vi "PID_Velocity.vi"() -> ()   [LabVIEW 2017]
uses:
  <vilib>/Platform/TimedLoop/XDataNode/timing_clust.ctl
  <vilib>/Platform/TimedLoop/XDataNode/nitl_modes.ctl
  <vilib>/Platform/TimedLoop/XDataNode/wakeup.ctl
  <vilib>/myRIO/Instrument Drivers/Onboard IO/AO/typedefs/AO Reference.ctl
  <vilib>/myRIO/Common/Instrument Driver Framework/Utilities/typedefs/myRIO Generic Hardware Reference.ctl
  <vilib>/myRIO/Common/Instrument Driver Framework/Utilities/typedefs/Hardware Version Enum.ctl
  <vilib>/myRIO/Common/Instrument Driver Framework/Utilities/typedefs/myRIO v1.0 Reference.ctl
  <vilib>/myRIO/Common/Instrument Driver Framework/Utilities/typedefs/Generic FPGA Reference.ctl
  <vilib>/myRIO/Common/Instrument Driver Framework/myRIO v1.0/AO/typedefs/AO Channels List.ctl
  <vilib>/myRIO/Common/Instrument Driver Framework/myRIO v1.0/AO/typedefs/AO Channels Enum.ctl
  <vilib>/myRIO/Common/Instrument Driver Framework/Utilities/typedefs/Analog Scaling Constants List.ctl
  <vilib>/myRIO/Common/Instrument Driver Framework/Utilities/typedefs/Analog Scaling Constants.ctl
  <vilib>/userdefined/High Color/nirio_resource_hc.ctl
  <vilib>/myRIO/Common/Instrument Driver Framework/Utilities/vis/Is FPGA Ref Available.vi
  <vilib>/myRIO/Common/Instrument Driver Framework/myRIO v1.0/AO/vis/myRIO v1.1 Open AO.vi
  <vilib>/myRIO/Instrument Drivers/Onboard IO/AO/vis/Write.vi
  <vilib>/myRIO/Common/Instrument Driver Framework/Utilities/vis/Validate Channels.vi
  <vilib>/myRIO/Common/Instrument Driver Framework/myRIO v1.0/AO/vis/myRIO v1.0 Reserve AO.vi
  <vilib>/myRIO/Common/Instrument Driver Framework/myRIO v1.0/AO/vis/myRIO v1.0 Build MUX Configuration AO.vi
  <vilib>/myRIO/Common/Instrument Driver Framework/myRIO v1.0/Resource Manager/vis/myRIO v1.0 Reserve Channel List.vi
  <vilib>/myRIO/Common/Instrument Driver Framework/myRIO v1.0/Resource Manager/vis/myRIO v1.0 Reserve Channel.vi
  <vilib>/myRIO/Common/Instrument Driver Framework/myRIO v1.0/Resource Manager/vis/myRIO v1.0 Unreserve Channel.vi
  <vilib>/myRIO/Common/Instrument Driver Framework/myRIO v1.0/Resource Manager/vis/myRIO v1.0 Build Mutex Name.vi
  <vilib>/Utility/VariantDataType/GetNumericInfo.vi
  <vilib>/Utility/error.llb/Error Cluster From Error Code.vi
  <vilib>/myRIO/Common/Instrument Driver Framework/myRIO v1.0/myRIO v1.1 Open.vi
  <vilib>/myRIO/Common/Instrument Driver Framework/myRIO v1.0/AO/vis/myRIO v1.0 Get Scaling Constants AO.vi
  <vilib>/myRIO/Common/Instrument Driver Framework/Utilities/vis/IO Manager.vi
  <vilib>/myRIO/Common/Instrument Driver Framework/Utilities/vis/Configuration Manager.vi
  <vilib>/myRIO/Common/Instrument Driver Framework/myRIO v1.0/myRIO v1.0 Close.vi
  <vilib>/myRIO/Common/Instrument Driver Framework/myRIO v1.0/AO/vis/myRIO v1.0 Write AO.vi
  <vilib>/addons/control/pid/pid.llb/PID (DBL).vi
  <vilib>/platform/TimedLoop/XDataNode/XDataNode.xnode
  <vilib>/myRIO/Express VI/Onboard IO/AO/AO Express VI.xnode
  <vilib>/myRIO/Instrument Drivers/Onboard IO/AO/vis/myRIO AO Open.xnode
  <vilib>/addons/control/pid/NI_PID_pid.lvlib
  <vilib>/myRIO/Instrument Drivers/Onboard IO/AO/AO.lvlib
  <vilib>/Platform/TimedLoop/XDataNode/XDNodeRunTimeDep.lvlib
panel:
  out "Velocity":dbl(graph)
  out "Theta Rate (deg/s)":dbl
  out "error out":errorcluster
  out "process variable":dbl
  out "Setpoint":dbl
  out "analog output":dbl format="%.2f"
  in  "PID Range":cluster{"output high":dbl, "output low":dbl}={"output high"=3.2, "output low"=1.8} {"output low" format="%.2f"; "output high" format="%.2f"}
  in  "PID gains":T1={"proportional gain (Kc)"=2.0, "integral time (Ti, min)"=0.05, "derivative time (Td, min)"=0.0} {"derivative time (Td, min)" format="%.3f"; "integral time (Ti, min)" format="%.3f"; "proportional gain (Kc)" format="%.3f"}
  out "Position":cluster{"setpoint":dbl, dbl}(graph)={"setpoint"=303.908879655711, 0.0}
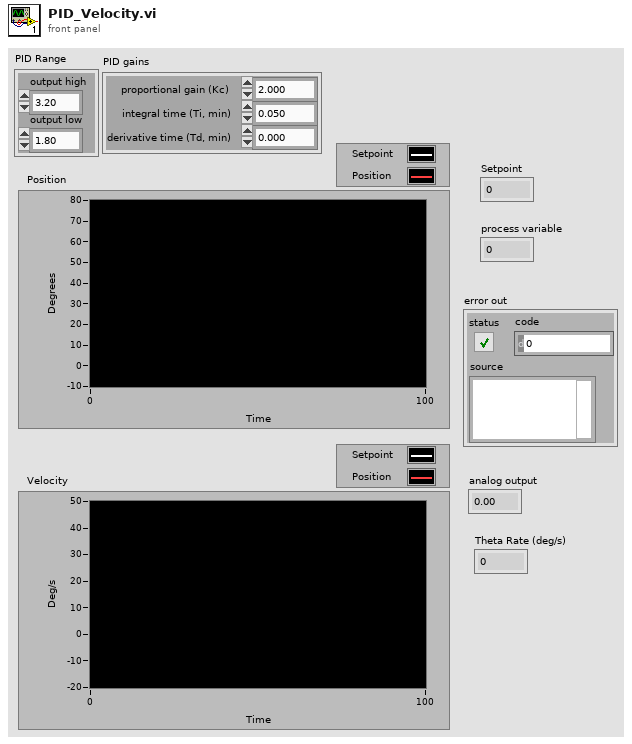
[diagram p1: front panel]
types:
  T1 = cluster{"proportional gain (Kc)":dbl, "integral time (Ti, min)":dbl, "derivative time (Td, min)":dbl}
  T2 = typedef "AO.lvlib/AO Reference.ctl" = cluster{"myRIO Reference":T3, "AO Channel List":T7, "AO Scaling Constant List":T9}
  T3 = typedef "myRIO Generic Hardware Reference.ctl" = cluster{"myRIO Model":T4, "myRIO Hardware Reference":T5}
  T4 = typedef "Hardware Version Enum.ctl" = enum16{"Unknown", "myRIO-1900", "myRIO-1950", "roboRIO", "NI ELVIS RIO CM"}
  T5 = typedef "myRIO v1.0 Reference.ctl" = cluster{"Generic FPGA Reference":T6, "Allow multiple opens":bool}
  T6 = typedef "Generic FPGA Reference.ctl" = refnum<k20>
  T7 = typedef "AO Channels List.ctl" = T8[]
  T8 = typedef "AO Channels Enum.ctl" = enum16{"Not Connected", "AudioOut/Left", "AudioOut/Right", "C/AO0", "C/AO1", "A/AO0", "A/AO1", "B/AO0", "B/AO1"}
  T9 = typedef "Analog Scaling Constants List.ctl" = T10[]
  T10 = typedef "Analog Scaling Constants.ctl" = cluster{"LSB Weight (Volts)":dbl, "Offset (Volts)":dbl, "Signed?":bool}
  T11 = typedef "nirio_resource_hc.ctl" = tag
  T12 = typedef "XDNodeRunTimeDep.lvlib/timing_clust.ctl" = cluster{"Expected End [f-1]":u64, "Actual End [f-1]":u64, "Finished Late? [f-1]":bool, "Expected End [i-1]":u64, "Actual End [i-1]":u64, "Finished Late? [i-1]":bool, "Expected Start [i]":u64, "Actual Start [i]":u64, "Expected Start [f]":u64, "Actual Start [f]":u64, "Source Name":string, "Structure Name":string, "Period":i64, "Deadline":i64, "Offset":i64, "Start":i64, "Priority":i32, "Timeout":i32, "Mode":T13, "Wakeup Reason":T14, "Error":errorcluster, "Source Type":string, "Secondary Source Type":string, "Global End Time":u64, "Global Start Time":u64, "Frame Duration":u64, "Iteration Duration":u64, "Assigned CPU":i32, "I/O Scan Engine Mode":u32}
  T13 = typedef "XDNodeRunTimeDep.lvlib/nitl_modes.ctl" = enum32{"No Change", "Process missed periods, maintain original phase", "Discard missed periods, maintain original phase", "Process missed periods, ignore original phase", "Discard missed periods, ignore original phase"}
  T14 = typedef "XDNodeRunTimeDep.lvlib/wakeup.ctl" = enum32{"Normal", "Aborted", "Asynchronous wakeup", "Timing source error", "Timed loop error", "Timeout"}
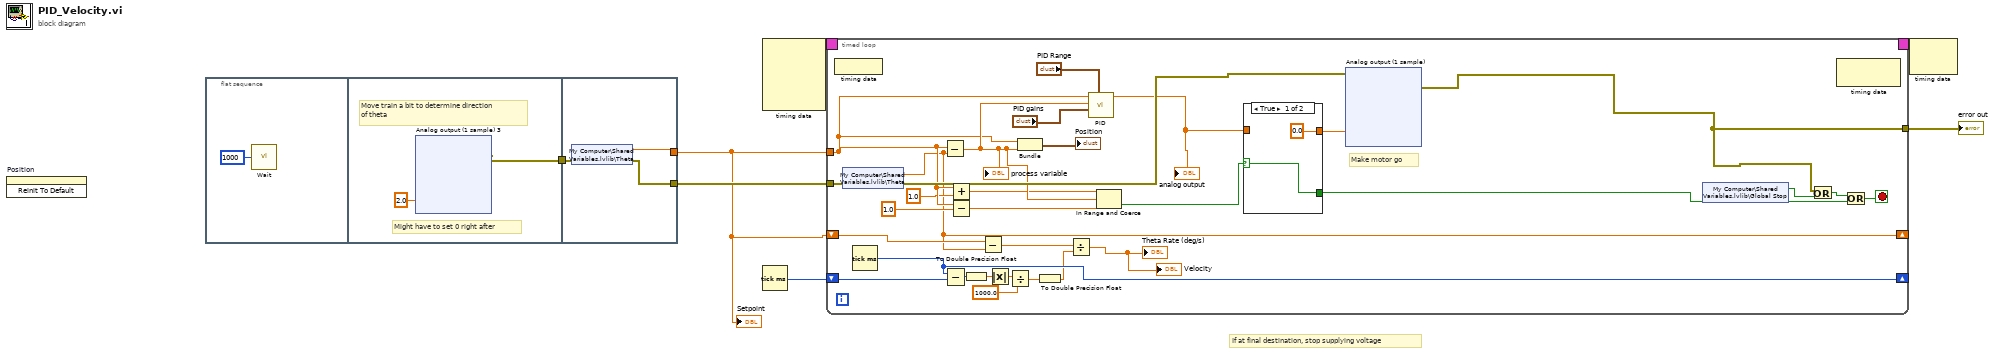
[diagram p0: block diagram]
diagram:
  # "If at final destination, stop supplying voltage"
  n1 = invoke on="Position" class="WFChart (strict)" method="Reinit To Default"() -> ()  [unwired: 3 in, 3 out]
  n2 = flat-sequence {
    tunnel: [w9] -> w3
    tunnel: [w50] -> w2
    tunnel: [w49] -> w5
    tunnel: w3 -> [w48]
    frame #0 {
      n3 = call "Wait"("Count(mSec)"=u32 1000) -> ()  [unwired: 1 out]
    }
    frame #1 {
      # "Might have to set 0 right after"
      # "Move train a bit to determine direction\nof theta"
      n4 = xnode "Analog output (1 sample) 3"("C/AO0 (AO0)"=2.0) -> ("error out"=w9:errorcluster)  [unwired: 1 in]
    }
    frame #2 {
      n5 = shared-variable "My Computer\\Shared Variables.lvlib\\Theta"(error in=w48) -> (w50:dbl, error out=w49:errorcluster)
    }
  }
  n6 = node-c288() -> (w7:T12)  [unwired: 4 in]
  n7 = Tick Count (ms)() -> (millisecond timer value=w1:u32)
  n8 = timed-loop {
    timing: w7 -> [_]
    timing-out: [_] -> w6
    tunnel: w2 -> [w75]
    tunnel: w5 -> [w78]
    tunnel: [w63] -> w4
    shift-right: [w51] -> _
    shift-left: w2 -> [w52]
    shift-right: [w61] -> _
    shift-left: w1 -> [w60]
    stop <- w65 stop-if-true
    # "Make motor go"
    n9 = node-c288() -> ()  [unwired: 1 in]
    n10 = shared-variable "My Computer\\Shared Variables.lvlib\\Theta"(error in=w78) -> (w51:dbl, error out=w77:errorcluster)
    n11 = Tick Count (ms)() -> (millisecond timer value=w61:u32)
    n12 = Subtract(x=w75, y=w51) -> (x-y=w76:dbl)
    "process variable" <- w76
    n13 = Subtract(x=w61, y=w60) -> (x-y=w56:u32)
    n14 = Add(x=w75, y=1.0) -> (x+y=w72:dbl)
    n15 = Subtract(x=w75, y=1.0) -> (x-y=w71:dbl)
    n16 = To Double Precision Float(number=w56) -> (double precision float=w55:dbl)
    n17 = Subtract(x=w52, y=w51) -> (x-y=w62:dbl)
    n18 = Absolute Value(x=w55) -> (abs(x)=w54:dbl)
    n19 = Divide(x=w54, y=1000.0) -> (x/y=w57:dbl)
    n20 = Bundle("Double"=w75, w76) -> (→"Position":cluster{"Double":dbl, dbl})  [unwired: 1 in]
    n21 = To Double Precision Float(number=w57) -> (double precision float=w59:dbl)
    n22 = Divide(x=w62, y=w59) -> (x/y=→"Theta Rate (deg/s)" →"Velocity":dbl)
    n23 = call-poly <vilib>:"PID.vi"("output range"="PID Range", "PID gains"="PID gains", "process variable"=w76, "setpoint"=w75) -> ("output"=w69:dbl)  [unwired: 6 in, 1 out]
    "analog output" <- w69
    n24 = In Range and Coerce(upper limit=w72, x=w76, lower limit=w71) -> (In Range?=w70:bool)  [unwired: 1 out]
    n25 = case shown="True" w70 {
      selector: w70 -> [w82 w84]
      tunnel: [0.0 ("output") w85] -> w68
      tunnel: w69 -> [_ w85]
      tunnel: [w82 w84] -> w67
      frame True {
      }
      frame False {
      }
    }
    n26 = xnode "Analog output (1 sample)"("C/AO0 (AO0)"=w68, "error in (no error)"=w77) -> ("error out"=w63:errorcluster)
    n27 = shared-variable "My Computer\\Shared Variables.lvlib\\Global Stop"() -> (w64:bool)  [unwired: 1 in, 1 out]
    n28 = Or(x=w63, y=w64) -> (x .or. y?=w66:bool)
    n29 = node-c288() -> ()  [unwired: 1 in, 1 out]
    n30 = Or(x=w66, y=w67) -> (x .or. y?=w65:bool)
  }
  "error out" <- w4
  n31 = node-c288(w6) -> ()  [unwired: 1 out]
  "Setpoint" <- w2
